vi "Send TCP_IP Message.vi"(8 "error in (no error)":errorcluster, 9 "timeout ms (25000)":u32=25000, 10 "Message":string, 11 "WebSocket in":refnum<class "WebSocket.lvclass">) -> (0 "error out":errorcluster, 3 "WebSocket out":refnum<class "WebSocket.lvclass">)   [LabVIEW 2024, in "Ramses Framework.lvlib"]
doc: "Appends a message size header to a message and sends it over TCP/IP"
uses:
  Ramses Framework.lvlib
  <vilib>/MediaMongrels Ltd/WebSockets/WebSockets/WebSocket/WebSocket.lvclass
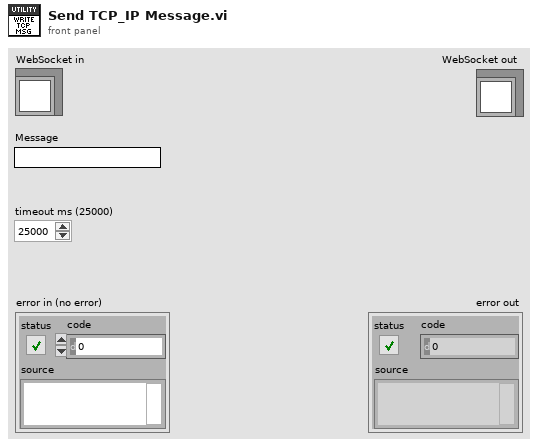
[diagram p1: front panel]
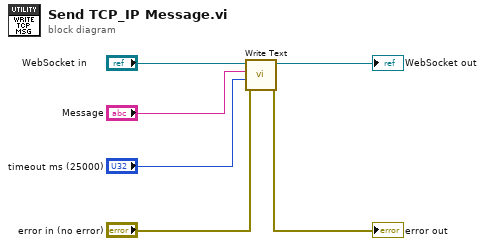
[diagram p0: block diagram]
diagram:
  n1 = call-dynamic "Write Text.vi"("error in (no error)"="error in (no error)", "timeout ms (5000)"="timeout ms (25000)", "String Data"="Message", "WebSocket in"="WebSocket in") -> ("error out"=→"error out":errorcluster, "WebSocket out"=→"WebSocket out":refnum<class "WebSocket.lvclass">)  [unwired: 6 in]
